vi "Save_double_Big_Array_to_Excel_Simple.vi"(6 "format string (%.3f)":string="%.3f" caption="포맷 문자열(%.3f)", 8 "에러 입력(에러 없음)":errorcluster, 9 "start (0, 0)":cluster{"row":i32, "column":i32}, 10 "배열":dbl[](array[numeric]) format="%#_9g", 11 "NI_report 입력":refnum<class "NI_report.lvclass">) -> (0 "error out":errorcluster, 1 "Next Position":cluster{"row":i32, "column":i32}, 3 "report out":refnum<class "NI_report.lvclass">)   [LabVIEW 2015]
uses:
  <vilib>/Utility/NIReport.llb/NI_report.lvclass
  <vilib>/Utility/NIReport.llb/Append Numeric Table to Report (wrap).vi
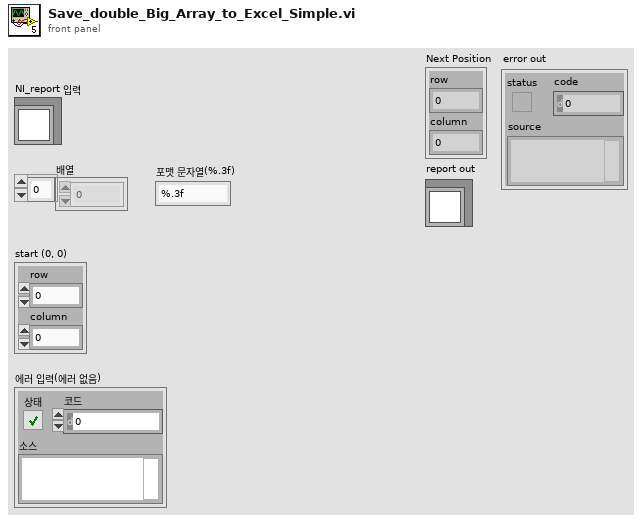
[diagram p1: front panel]
types:
  T1 = cluster{"position (excel)":cluster{"row":i32, "column":i32}, "name (excel)":string, "bookmark (word)":string}
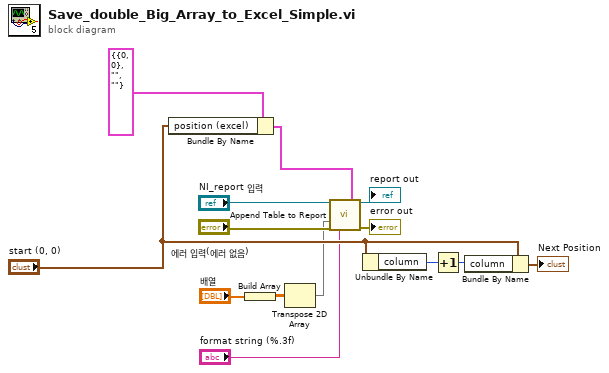
[diagram p0: block diagram]
diagram:
  n1 = Bundle By Name(cluster=T1 {"position (excel)"={"row"=0, "column"=0}, "name (excel)"="", "bookmark (word)"=""} ("MS Office parameters"), "position (excel)"="start (0, 0)") -> (w4:T1)
  n2 = Build Array("배열") -> (w6:dbl[][])
  n3 = Transpose 2D Array(2D array=w6) -> (transposed array=w2:dbl[][])
  n4 = call-poly <vilib>:"Append Table to Report.vi"("report in"="NI_report 입력", "MS Office parameters"=w4, "numerical data"=w2, "error in (no error)"="에러 입력(에러 없음)", "format string (%.3f)"="format string (%.3f)") -> ("report out"=→"report out":refnum<class "NI_report.lvclass">, "error out"=→"error out":errorcluster)  [unwired: 7 in, 2 out]
  n5 = Unbundle By Name("start (0, 0)") -> ("column"=w13:i32)
  n6 = Increment(x=w13) -> (x+1=w14:i32)
  n7 = Bundle By Name(cluster="start (0, 0)", "column"=w14) -> (→"Next Position":cluster{"row":i32, "column":i32})
